vi "Settings Dialog.vi"(8 "error in (no error)":errorcluster, 9 "UI State":T1, 10 "Message Queues":T2, 11 "PRM State Cluster In":T6={"PRM Config"={"GUID"="", "Drop Coords"={"Horizontal"=0, "Vertical"=0}, "Process Name"="", "Settings"={"Cycle Period"=500.0, "PID 2 Parameters"={"Input Device"=enum."Default", "Output Device"=enum."Default", "Setpoint"=0.0, "PID gains"={"proportional gain (Kc)"=1.0, "integral time (Ti, min)"=0.01, "derivative time (Td, min)"=0.0}, "output range"={"output low"=0.0, "output high"=100.0}}, "Manual Entry"=0.0, "Auto?"=TRUE, "4-20mA Input Settings"={"Input Channel "=0}, "4-20mA Out Settings"={"Output DAQ Task"=""}, "Input Channel Tag Name "=""}, "Settings Load Count"=0}, "State"=enum."Idle", "Start Time"=timestamp(0 s since 1904-01-01), "Current Time"=timestamp(0 s since 1904-01-01), "First Iteration"=FALSE, "Data"={"4-20mA Input"=0.0, "PID 2 Process Variable"=0.0, "PID 2 Output"=0.0, "4-20mA Output"=0.0}} {"PRM Config"."Settings"."PID 2 Parameters"."output range"."output low" format="%.2f"; "PRM Config"."Settings"."PID 2 Parameters"."output range"."output high" min=0.0 max=100.0 format="%.2f"; "PRM Config"."Settings"."PID 2 Parameters"."PID gains"."derivative time (Td, min)" format="%.3f"; "PRM Config"."Settings"."PID 2 Parameters"."PID gains"."integral time (Ti, min)" format="%.3f"; "PRM Config"."Settings"."PID 2 Parameters"."PID gains"."proportional gain (Kc)" format="%.3f"}) -> (0 "error out":errorcluster, 1 "Cancelled?":bool=TRUE, 2 "UI Refresh Needed?":bool, 3 "PRM State Cluster Out":T6={"PRM Config"={"GUID"="", "Drop Coords"={"Horizontal"=0, "Vertical"=0}, "Process Name"="", "Settings"={"Cycle Period"=500.0, "PID 2 Parameters"={"Input Device"=enum."Default", "Output Device"=enum."Default", "Setpoint"=0.0, "PID gains"={"proportional gain (Kc)"=1.0, "integral time (Ti, min)"=0.01, "derivative time (Td, min)"=0.0}, "output range"={"output low"=0.0, "output high"=100.0}}, "Manual Entry"=0.0, "Auto?"=TRUE, "4-20mA Input Settings"={"Input Channel "=0}, "4-20mA Out Settings"={"Output DAQ Task"=""}, "Input Channel Tag Name "=""}, "Settings Load Count"=0}, "State"=enum."Idle", "Start Time"=timestamp(0 s since 1904-01-01), "Current Time"=timestamp(0 s since 1904-01-01), "First Iteration"=FALSE, "Data"={"4-20mA Input"=0.0, "PID 2 Process Variable"=0.0, "PID 2 Output"=0.0, "4-20mA Output"=0.0}} {"PRM Config"."Settings"."PID 2 Parameters"."output range"."output low" format="%.2f"; "PRM Config"."Settings"."PID 2 Parameters"."output range"."output high" min=0.0 max=100.0 format="%.2f"; "PRM Config"."Settings"."PID 2 Parameters"."PID gains"."derivative time (Td, min)" format="%.3f"; "PRM Config"."Settings"."PID 2 Parameters"."PID gains"."integral time (Ti, min)" format="%.3f"; "PRM Config"."Settings"."PID 2 Parameters"."PID gains"."proportional gain (Kc)" format="%.3f"})   [LabVIEW 2018, in "4-20mA Module.lvlib"]
uses:
  4-20mA Module.lvlib
  Controls/4-20mA Module State Cluster.ctl
  Controls/4-20mA Module Config Cluster.ctl
  <vilib>/Utility/miscctls.llb/LVPoint32TypeDef.ctl
  Controls/4-20mA Module Settings Cluster.ctl
  Pressure Transmitter/Pressure Transmitter Device Settings.ctl
  Pressure Reg Module/Pressure Regulator Device Settings.ctl
  Measure Instrument/State Enum.ctl
  Controls/4-20mA Message Queues.ctl
  support/Message Queue/Message Cluster.ctl
  controls/UI State.ctl
  Tag VIs/Tag FGV Operation Enum.ctl
  <vilib>/Utility/miscctls.llb/LVMinMaxIncTypeDef.ctl
  support/Message Queue/Enqueue Message (Single).vi
  Settings/Settings.lvlib
  Pressure Transmitter/Pressure Transmitter Library.lvlib
  Shared Variables/Dynamic Shared Variables.lvlib
  Pressure Reg Module/Pressure Regulator Library.lvlib
  support/Support Library.lvlib
  support/Message Queue/Message Queue.lvlib
  Flow Regulator/Pressure Reg Module/Flow Regulator Library.lvlib
  <vilib>/Utility/xml.llb/Write to XML File(string).vi
  Measure Instrument/Feed Module Engine.lvlib
panel:
  in  "Module Name":string
  in  "Start":bool
  in  "Stop":bool
  in  "Pressure Regulator Configuration":T5={"Cycle Period"=500.0, "PID 2 Parameters"={"Input Device"=enum."Default", "Output Device"=enum."Default", "Setpoint PSIA"=0.0, "PID gains"={"proportional gain (Kc)"=1.0, "integral time (Ti, min)"=0.01, "derivative time (Td, min)"=0.0}, "output range"={"output low"=0.0, "output high"=100.0}}, "Manual PSIA"=0.0, "Auto?"=TRUE, "4-20mA Input Settings"={"Input Channel "=0}, "Out Settings"={"Output DAQ Task"=""}} {"4-20mA Input Settings"."Input Channel" items=["Default", "TT0", "PT0", "PR 1:4-20mA Input", "PR 1:PID2Out", "PR 1:4-20mA Output", "PR 1:Input Device Disconnected", "PR 1:Output Device Disconnected"]; "Manual PSIA" min=0.0 max=50.0; "PID 2 Parameters"."output range"."output low" format="%.2f"; "PID 2 Parameters"."output range"."output high" min=0.0 max=100.0 format="%.2f"; "PID 2 Parameters"."PID gains"."derivative time (Td, min)" format="%.3f"; "PID 2 Parameters"."PID gains"."integral time (Ti, min)" format="%.3f"; "PID 2 Parameters"."PID gains"."proportional gain (Kc)" format="%.3f"}
  in  "Cancel Button":bool
  in  "OK Button":bool
  # "Output Settings"
  # "Input Settings"
  # "Instrument Settings"
  # "Instrument Settings"
  # "Instrument Settings"
  # "Instrument Settings"
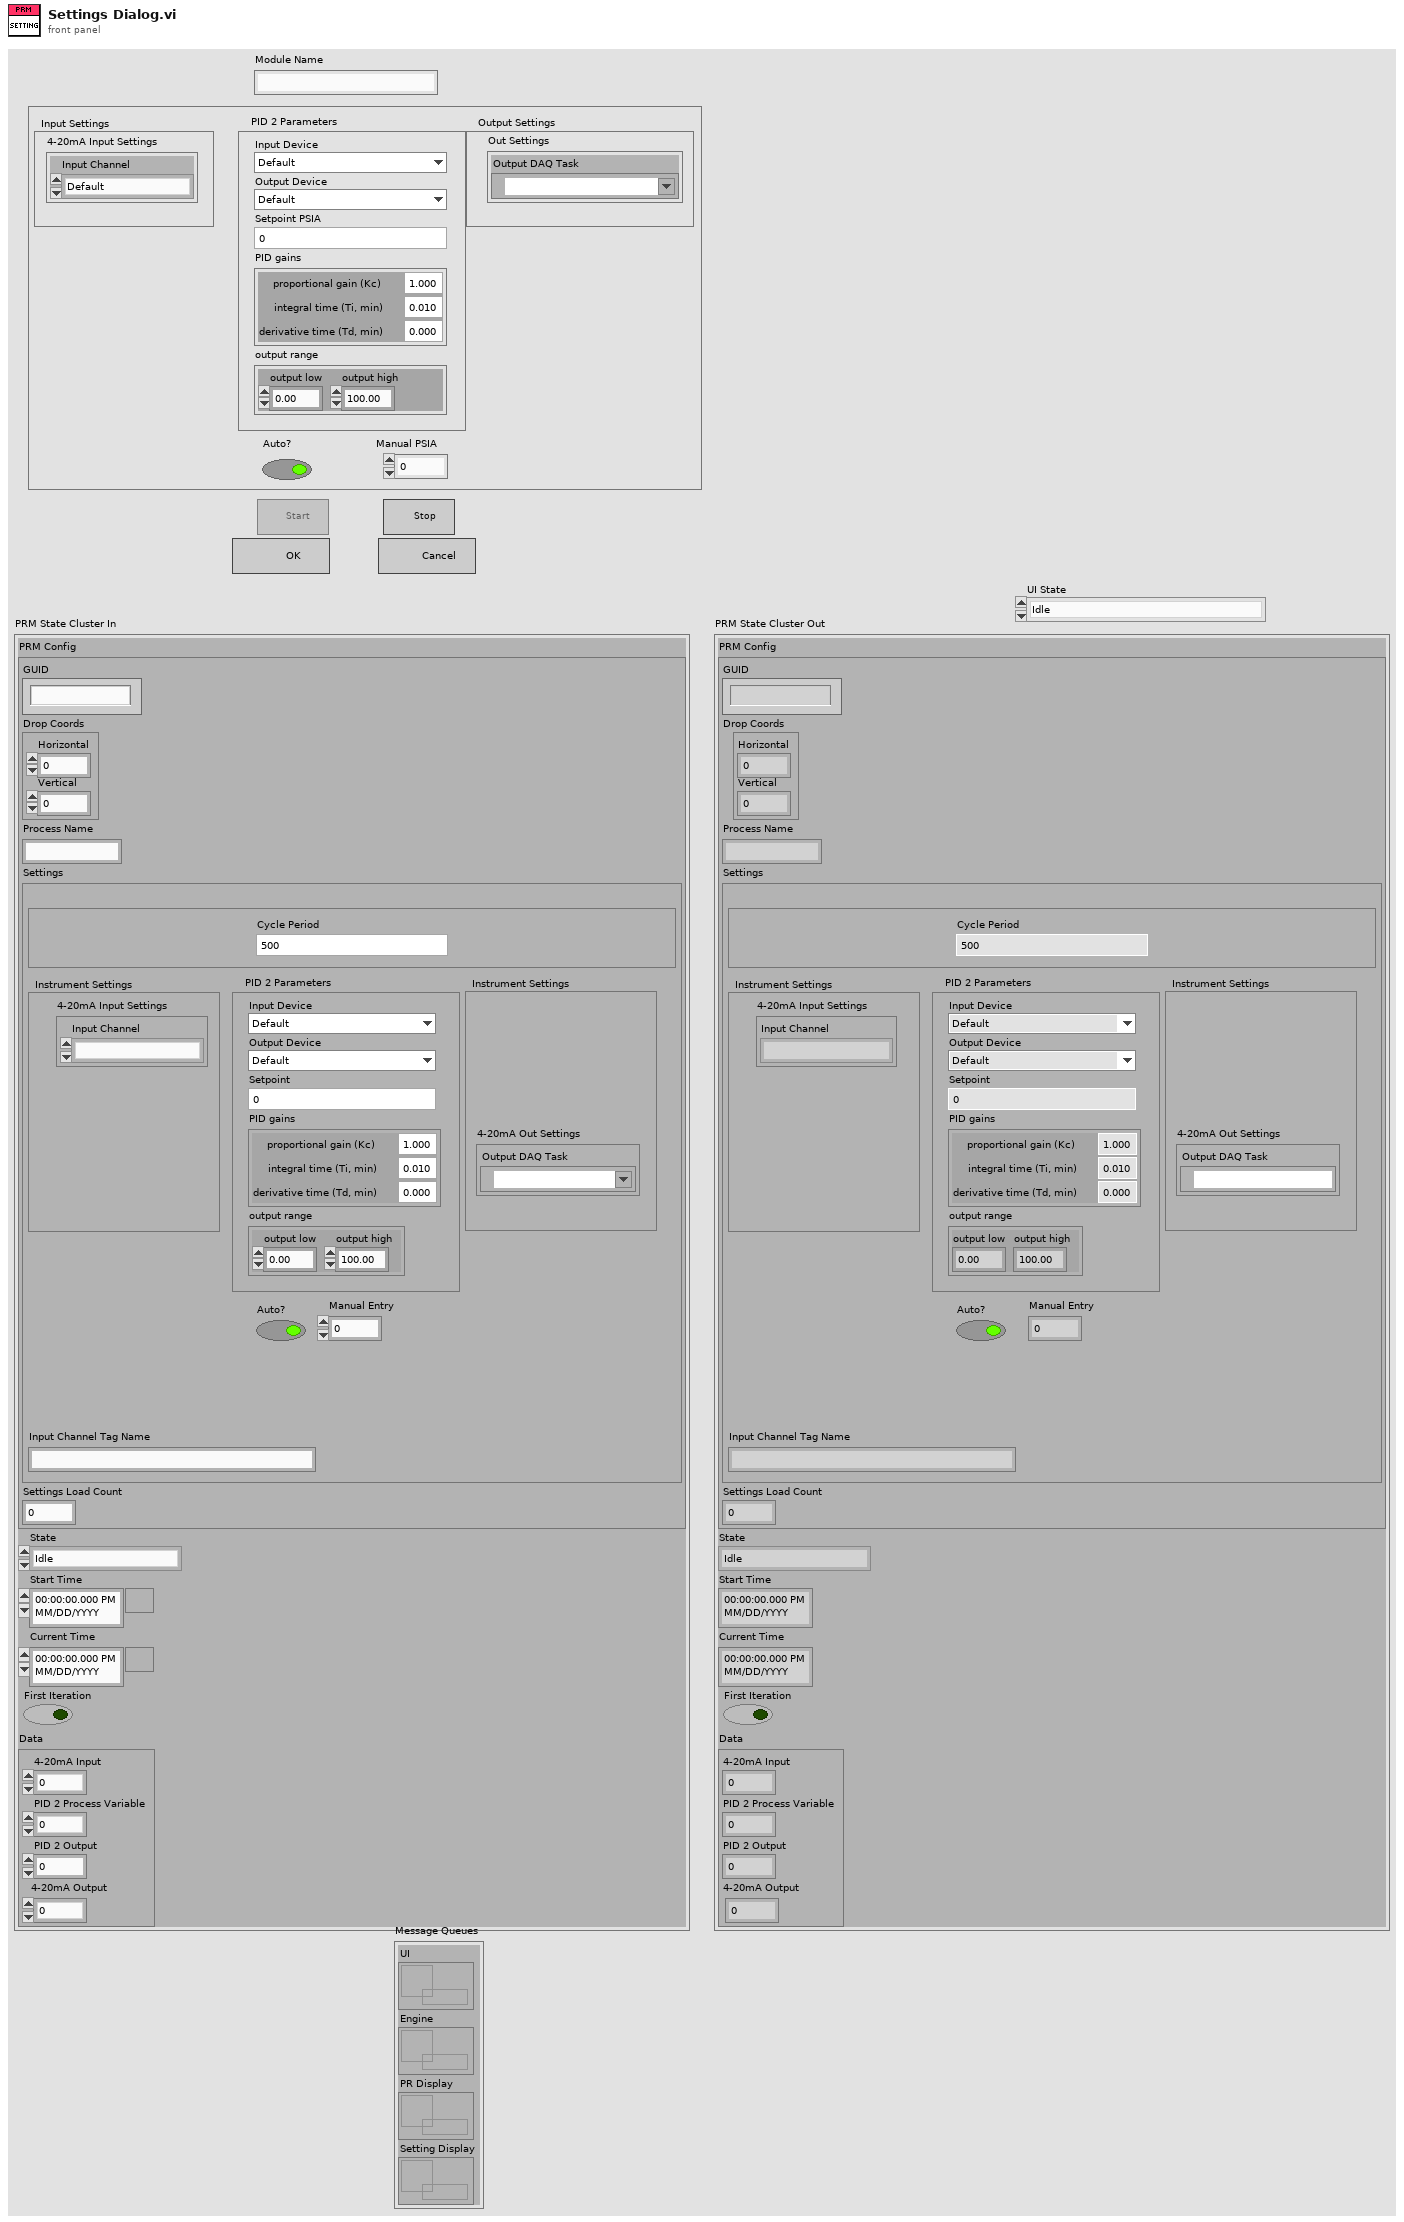
[diagram p1: front panel]
types:
  T1 = typedef "UI State.ctl" = enum16{"Idle", "Acquiring and Logging", "Waiting for Exit", "Waiting for Exit (Acq Stopped)", "Waiting for Exit (Log Stopped)", "Waiting for Stop", "Waiting for Stop (Acq Stopped)", "Waiting for Stop (Log Stopped)"}
  T2 = typedef "4-20mA Module.lvlib/4-20mA Message Queues.ctl" = cluster{"UI":refnum<queue>, "Engine":refnum<queue>, "PR Display":refnum<queue>, "Setting Display":refnum<queue>}
  T3 = typedef "Pressure Transmitter Library.lvlib/Pressure Transmitter Device Settings.ctl" = cluster{"Input Channel ":u16}
  T4 = typedef "Pressure Regulator Library.lvlib/Pressure Regulator Device Settings.ctl" = cluster{"Output DAQ Task":refnum<k21>}
  T5 = cluster{"Cycle Period":dbl, "PID 2 Parameters":cluster{"Input Device":enum16{"Default", "4-20mA"}, "Output Device":enum16{"Default", "Equilibar Pressure Reg", "Flow Regulator"}, "Setpoint PSIA":dbl, "PID gains":cluster{"proportional gain (Kc)":dbl, "integral time (Ti, min)":dbl, "derivative time (Td, min)":dbl}, "output range":cluster{"output low":dbl, "output high":dbl}}, "Manual PSIA":dbl, "Auto?":bool, "4-20mA Input Settings":T3, "Out Settings":T4}
  T6 = typedef "4-20mA Module.lvlib/4-20mA Module State Cluster.ctl" = cluster{"PRM Config":T7, "State":T10, "Start Time":timestamp, "Current Time":timestamp, "First Iteration":bool, "Data":cluster{"4-20mA Input":dbl, "PID 2 Process Variable":dbl, "PID 2 Output":dbl, "4-20mA Output":dbl}}
  T7 = typedef "4-20mA Module.lvlib/4-20mA Module Config Cluster.ctl" = cluster{"GUID":string, "Drop Coords":T8, "Process Name":string, "Settings":T9, "Settings Load Count":i32}
  T8 = typedef "LVPoint32TypeDef.ctl" = cluster{"Horizontal":i32, "Vertical":i32}
  T9 = typedef "4-20mA Module.lvlib/4-20mA Module Settings Cluster.ctl" = cluster{"Cycle Period":dbl, "PID 2 Parameters":cluster{"Input Device":enum16{"Default", "4-20mA"}, "Output Device":enum16{"Default", "Equilibar Pressure Reg", "Flow Regulator"}, "Setpoint":dbl, "PID gains":cluster{"proportional gain (Kc)":dbl, "integral time (Ti, min)":dbl, "derivative time (Td, min)":dbl}, "output range":cluster{"output low":dbl, "output high":dbl}}, "Manual Entry":dbl, "Auto?":bool, "4-20mA Input Settings":T3, "4-20mA Out Settings":T4, "Input Channel Tag Name ":string}
  T10 = typedef "Feed Module.lvlib/Feed Module Engine.lvlib/State Enum.ctl" = enum16{"Measuring", "Idle", "Paused"}
  T11 = typedef "Tag FGV Operation Enum.ctl" = enum16{"Init", "Set Notification Queue", "Create Tag", "Commit", "Write Tag (Numeric)", "Write Tag (Boolean)", "Read All Tags", "Read One Tag", "Delete Tag Category", "Set Alarm Parameters (Numeric)", "Set Alarm Parameters (Boolean)", "Enable All Alarms", "Disable All Alarms", "Delete All Tags", "Read Alarms", "Ack Alarm"}
  T12 = enum8{"Enabled", "Disabled", "Disabled and Grayed Out"}
  T13 = cluster{"Cycle Period":dbl, "PID 2 Parameters":cluster{"Input Device":enum16{"Default", "4-20mA"}, "Output Device":enum16{"Default", "Equilibar Pressure Reg", "Flow Regulator"}, "Setpoint":dbl, "PID gains":cluster{"proportional gain (Kc)":dbl, "integral time (Ti, min)":dbl, "derivative time (Td, min)":dbl}, "output range":cluster{"output low":dbl, "output high":dbl}}, "Manual Entry":dbl, "Auto?":bool, "4-20mA Input Settings":T3, "Out Settings":T4}
  T14 = typedef "LVMinMaxIncTypeDef.ctl" = cluster{"Minimum":dbl, "Maximum":dbl, "Increment":dbl}
  T15 = cluster{"Input Device":enum16{"Default", "4-20mA"}, "Output Device":enum16{"Default", "Equilibar Pressure Reg", "Flow Regulator"}, "Setpoint":dbl, "PID gains":cluster{"proportional gain (Kc)":dbl, "integral time (Ti, min)":dbl, "derivative time (Td, min)":dbl}, "output range":cluster{"output low":dbl, "output high":dbl}}
  T16 = cluster{"Input Device":enum16{"Default", "4-20mA"}, "Output Device":enum16{"Default", "Equilibar Pressure Reg", "Flow Regulator"}, "Setpoint PSIA":dbl, "PID gains":cluster{"proportional gain (Kc)":dbl, "integral time (Ti, min)":dbl, "derivative time (Td, min)":dbl}, "output range":cluster{"output low":dbl, "output high":dbl}}
  T17 = enum16{"Default", "Equilibar Pressure Reg", "Flow Regulator"}
  T18 = cluster{"Numeric Text.Text":dbl, "Numeric Text.Text":dbl, "Numeric Text.Text":dbl}
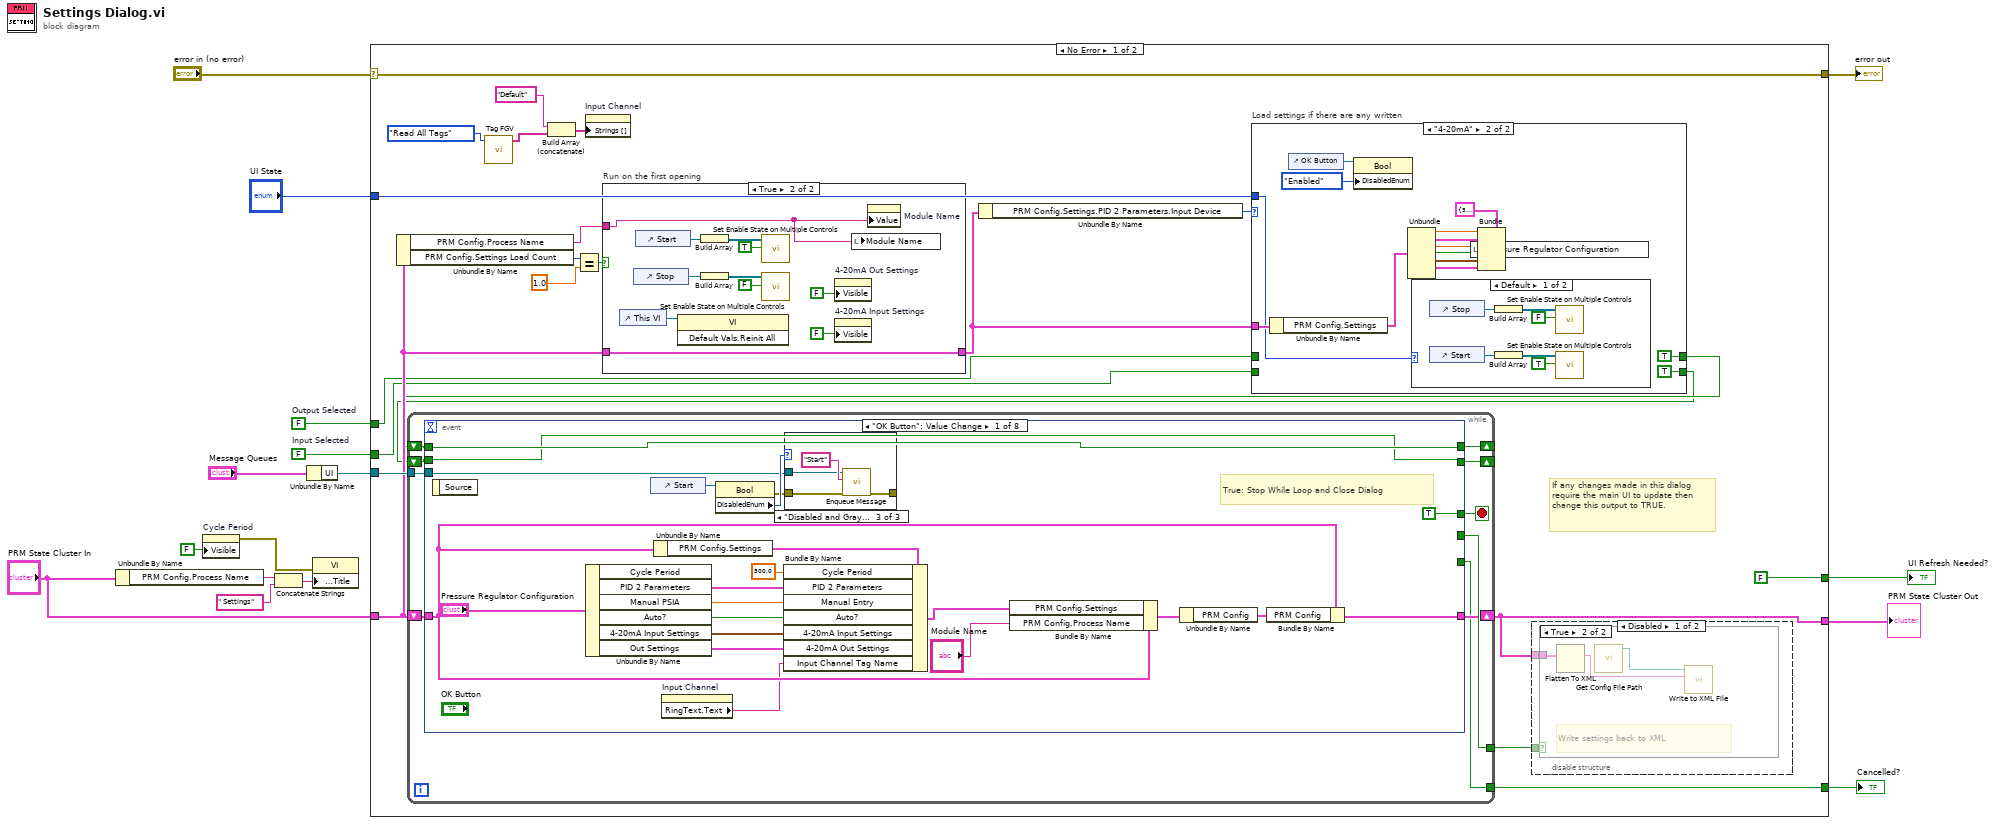
[diagram p0: block diagram]
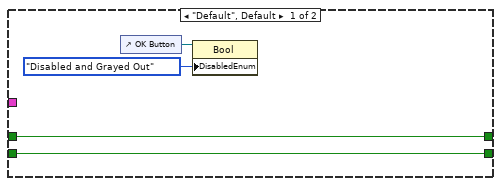
[diagram p4: hidden frame]
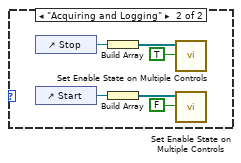
[diagram p5: hidden frame]
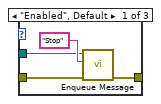
[diagram p7: hidden frame]
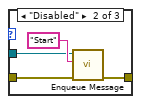
[diagram p8: hidden frame]
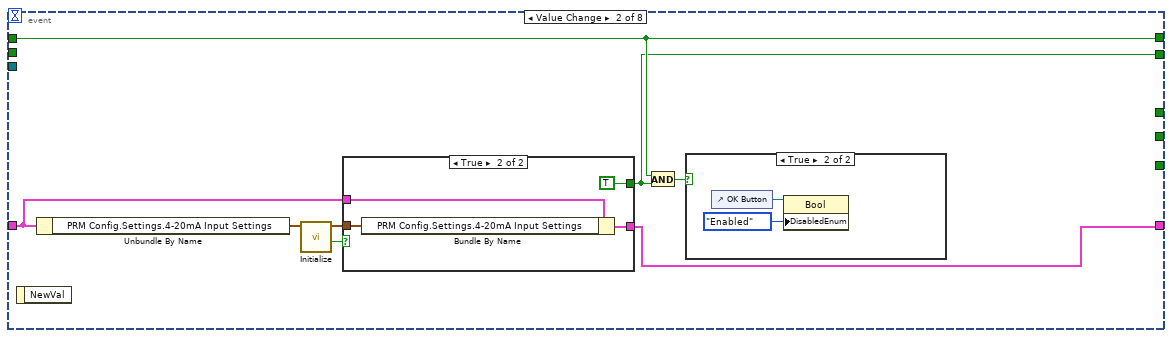
[diagram p9: hidden frame]
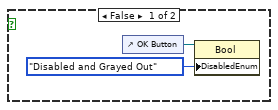
[diagram p10: hidden frame]
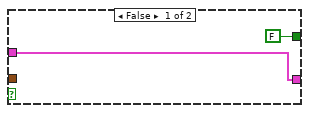
[diagram p11: hidden frame]
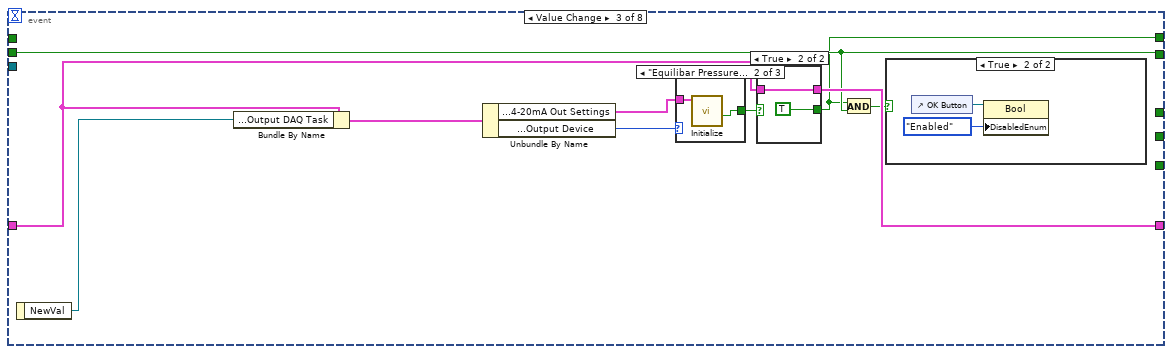
[diagram p12: hidden frame]
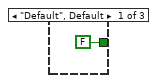
[diagram p13: hidden frame]
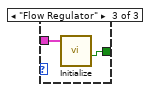
[diagram p14: hidden frame]
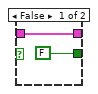
[diagram p15: hidden frame]
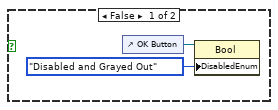
[diagram p16: hidden frame]
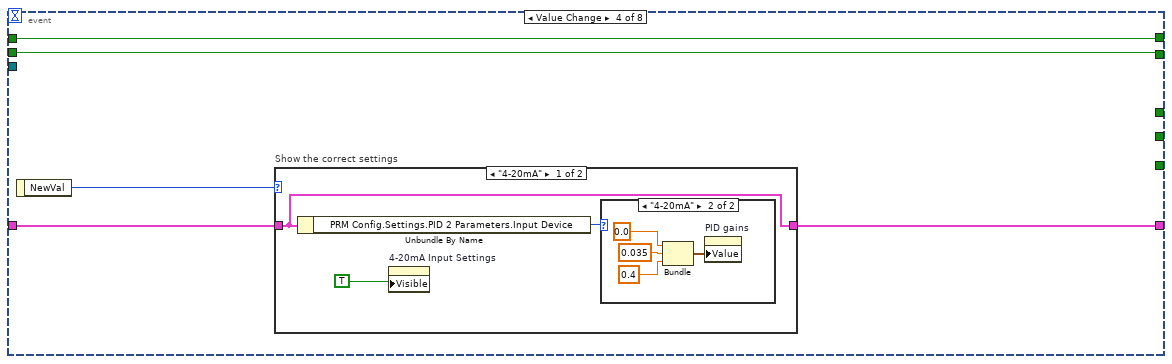
[diagram p17: hidden frame]
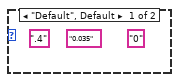
[diagram p18: hidden frame]
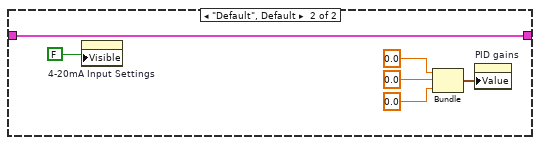
[diagram p19: hidden frame]
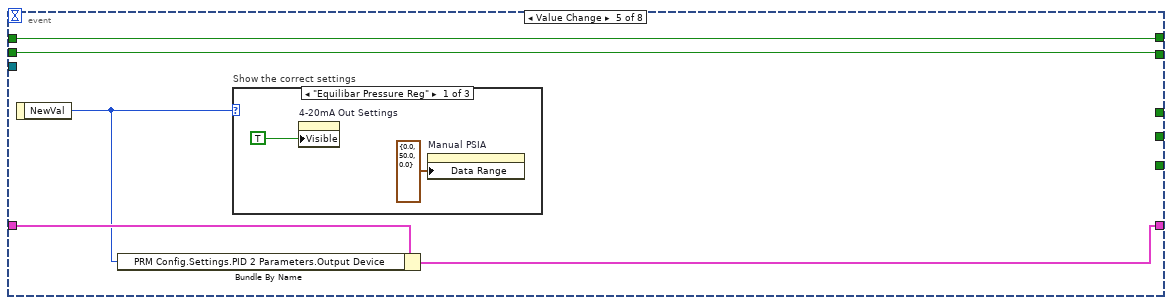
[diagram p20: hidden frame]
diagram:
  w5 = FALSE  # Input Selected
  w6 = FALSE  # Output Selected
  n1 = Unbundle By Name("PRM State Cluster In") -> ("PRM Config.Process Name"=w13:string)
  n2 = property on="Cycle Period" class="DigNum (strict)"("Visible"=FALSE) -> (error out=w1:errorcluster)  [unwired: 2 in, 1 out]
  n3 = Concatenate Strings(w13, " Settings" ("string")) -> (w12:string)
  n4 = Unbundle By Name("Message Queues") -> ("UI"=w7:refnum<queue>)
  n5 = property class="VI"(error in=w1, "Front Panel.Title"=w12) -> ()  [unwired: 1 in, 2 out]
  n6 = case shown="No Error" "error in (no error)" {
    selector: "error in (no error)" -> [w38 w231]
    tunnel: [w38 w231] -> w16
    tunnel: "PRM State Cluster In" -> [w23 w230]
    tunnel: [w36 w230] -> w10
    tunnel: [FALSE ("UI Refresh Needed?") _] -> w15
    tunnel: [w35 TRUE ("UI Refresh Needed?")] -> w14
    tunnel: w7 -> [w24 _]
    tunnel: w6 -> [w22 _]
    tunnel: w5 -> [w21 _]
    tunnel: "UI State" -> [w18 _]
    frame No Error {
      # "If any changes made in this dialog require the main UI to update then change this output to TRUE."
      n7 = Unbundle By Name(w23) -> ("PRM Config.Process Name"=w17:string, "PRM Config.Settings Load Count"=w34:i32)
      n8 = call "Tag FGV.vi"("Operation"=Tag_FGV_Operation_Enum."Read All Tags") -> ("Tag Names"=w26:string[])  [unwired: 5 in, 5 out]
      n9 = Build Array (concatenate)("Default", w26) -> (w25:string[])
      n10 = Equal?(x=w34, y=1.0) -> (x = y?=w31:bool)
      n11 = property on="Input Channel" class="Ring (strict)"("Strings []"=w25) -> ()  [unwired: 2 in, 2 out]
      n12 = case "Run on the first opening" shown="True" w31 {
        tunnel: w23 -> [w75 w85]
        tunnel: [w75 w85] -> w29
        tunnel: w17 -> [_ w76]
        frame False {
        }
        frame True {
          n13 = control-ref of="This VI"() -> (w86:refnum<vi>)
          n14 = control-ref of="Stop"() -> (w81:refnum<vi>)
          n15 = control-ref of="Start"() -> (w82:refnum<vi>)
          n16 = invoke class="VI" method="Default Vals.Reinit All"(reference=w86) -> ()  [unwired: 2 in, 3 out]
          n17 = Build Array(w82) -> (w80:refnum<vi>[])
          n18 = Build Array(w81) -> (w79:refnum<vi>[])
          n19 = call "Set Enable State on Multiple Controls.vi"("Enable?"=TRUE, "Controls"=w80) -> ()  [unwired: 10 in]
          n20 = call "Set Enable State on Multiple Controls.vi"("Enable?"=FALSE, "Controls"=w79) -> ()  [unwired: 10 in]
          n21 = property on="4-20mA Out Settings" class="Clust (strict)"("Visible"=FALSE) -> ()  [unwired: 2 in, 2 out]
          n22 = property on="4-20mA Input Settings" class="Clust (strict)"("Visible"=FALSE) -> ()  [unwired: 2 in, 2 out]
          n23 = local write "Module Name"(w76) -> ()
          n24 = property on="Module Name" class="Str"("Value"=w76) -> ()  [unwired: 2 in, 2 out]
        }
      }
      n25 = Unbundle By Name(w29) -> ("PRM Config.Settings.PID 2 Parameters.Input Device"=w30:enum16{"Default", "4-20mA"})
      n26 = case "Load settings if there are any written" shown="\"4-20mA\"" w30 {
        tunnel: w29 -> [_ w56]
        tunnel: w22 -> [w45 _]
        tunnel: w21 -> [w44 _]
        tunnel: [w45 TRUE] -> w20
        tunnel: [w44 TRUE] -> w19
        tunnel: w18 -> [_ w48]
        frame "Default", Default {
          n27 = control-ref of="OK Button"() -> (w47:refnum<vi>)
          n28 = property on="Property Node" class="Bool"(reference=w47, "DisabledEnum"=T12."Disabled and Grayed Out" ("Disabled")) -> ()  [unwired: 1 in, 2 out]
        }
        frame "4-20mA" {
          n29 = Unbundle By Name(w56) -> ("PRM Config.Settings"=w60:T9)
          n30 = control-ref of="OK Button"() -> (w54:refnum<vi>)
          n31 = property on="Property Node" class="Bool"(reference=w54, "DisabledEnum"=T12."Enabled" ("Disabled")) -> ()  [unwired: 1 in, 2 out]
          n32 = Unbundle(w60) -> ("Cycle Period"=w61:dbl, "PID 2 Parameters"=w62:T15, "Manual Entry"=w57:dbl, "Auto?"=w58:bool, "4-20mA Input Settings"=w59:T3, "4-20mA Out Settings"=w52:T4)  [unwired: 1 out]
          n33 = case shown="Default" w48 {
            frame Default {
              n34 = control-ref of="Stop"() -> (w66:refnum<vi>)
              n35 = control-ref of="Start"() -> (w67:refnum<vi>)
              n36 = Build Array(w66) -> (w65:refnum<vi>[])
              n37 = Build Array(w67) -> (w68:refnum<vi>[])
              n38 = call "Set Enable State on Multiple Controls.vi"("Enable?"=FALSE, "Controls"=w65) -> ()  [unwired: 10 in]
              n39 = call "Set Enable State on Multiple Controls.vi"("Enable?"=TRUE, "Controls"=w68) -> ()  [unwired: 10 in]
            }
            frame "Acquiring and Logging" {
              n40 = control-ref of="Stop"() -> (w72:refnum<vi>)
              n41 = control-ref of="Start"() -> (w73:refnum<vi>)
              n42 = Build Array(w72) -> (w71:refnum<vi>[])
              n43 = Build Array(w73) -> (w74:refnum<vi>[])
              n44 = call "Set Enable State on Multiple Controls.vi"("Enable?"=TRUE, "Controls"=w71) -> ()  [unwired: 10 in]
              n45 = call "Set Enable State on Multiple Controls.vi"("Enable?"=FALSE, "Controls"=w74) -> ()  [unwired: 10 in]
            }
          }
          n46 = Bundle(cluster=T13 {"Cycle Period"=500.0, "PID 2 Parameters"={"Input Device"=enum."Default", "Output Device"=enum."Default", "Setpoint"=0.0, "PID gains"={"proportional gain (Kc)"=1.0, "integral time (Ti, min)"=0.01, "derivative time (Td, min)"=0.0}, "output range"={"output low"=0.0, "output high"=100.0}}, "Manual Entry"=0.0, "Auto?"=TRUE, "4-20mA Input Settings"={"Input Channel "=0}, "Out Settings"={"Output DAQ Task"=""}} ("Configuration"), "Cycle Period"=w61, "PID 2 Parameters"=w62, "Manual Entry"=w57, "Auto?"=w58, "4-20mA Input Settings"=w59, "Out Settings"=w52) -> (w55:T13)
          n47 = local write "Pressure Regulator Configuration"(w55) -> ()
        }
      }
      n48 = while {
        tunnel: [w96] -> w32
        tunnel: [w93] -> w35
        tunnel: w24 -> [w92]
        shift-right: [w88] -> _
        shift-left: w20 -> [w91]
        shift-right: [w89] -> _
        shift-left: w19 -> [w90]
        shift-right: [w95] -> w36
        shift-left: w23 -> [w87]
        stop <- w94 stop-if-true
        n49 = event shown="[0] \"OK Button\": Value Change" {
          selector: _ -> [_ _ _ _ _ _ _ _]
          dyn-events: _ -> [_ _ _ _ _ _ _ _]
          timeout: _ -> [_ _ _ _ _ _ _ _]
          tunnel: [w106 w140 w160 w178 w192 w202 w219 w228] -> w95
          tunnel: w87 -> [w107 w137 w154 w177 w194 w205 w219 w228]
          tunnel: [FALSE ("UI Refresh Needed?") _ _ _ _ FALSE ("UI Refresh Needed?") _ _] -> w96
          tunnel: [TRUE _ _ _ _ TRUE _ _] -> w94
          tunnel: [FALSE ("UI Refresh Needed?") _ _ _ _ TRUE ("UI Refresh Needed?") _ _] -> w93
          tunnel: w92 -> [w102 _ _ _ _ _ _ _]
          tunnel: w91 -> [w100 w134 _ w175 w196 w207 w212 w221]
          tunnel: w90 -> [w99 _ w156 w174 w195 w206 w211 w220]
          tunnel: [w99 w133 w156 w174 w195 w206 w211 w220] -> w89
          tunnel: [w100 w134 w152 w175 w196 w207 w212 w221] -> w88
          event "OK Button": Value Change {
            # "True: Stop While Loop and Close Dialog"
            n50 = event-data() -> ()  [unwired: 1 in, 1 out]
            n51 = Unbundle By Name("Pressure Regulator Configuration") -> ("PID 2 Parameters"=w116:T16, "Manual PSIA"=w115:dbl, "Auto?"=w114:bool, "4-20mA Input Settings"=w112:T3, "Out Settings"=w111:T4)  [unwired: 1 out]
            n52 = control-ref of="Start"() -> (w101:refnum<vi>)
            n53 = Unbundle By Name(w107) -> ("PRM Config.Settings"=w110:T9)
            n54 = property on="Input Channel" class="Ring (strict)"() -> ("RingText.Text"=w105:string)  [unwired: 2 in, 2 out]
            n55 = property class="Bool"(reference=w101) -> (error out=w103:errorcluster, "DisabledEnum"=w104:T12)  [unwired: 1 in, 1 out]
            n56 = Bundle By Name(cluster=w110, "Cycle Period"=500.0, "PID 2 Parameters"=w116, "Manual Entry"=w115, "Auto?"=w114, "4-20mA Input Settings"=w112, "4-20mA Out Settings"=w111, "Input Channel Tag Name"=w105) -> (w113:T9)
            n57 = case shown="\"Disabled and Grayed Out\"" w104 {
              tunnel: w103 -> [w122 w127 w131]
              tunnel: [w124 w126 w130] -> _
              tunnel: w102 -> [w121 w125 w129]
              frame "Enabled", Default {
                n58 = call-poly "Enqueue Message.vi"("error in (no error)"=w122, "Message"="Stop", "Message Queue"=w121) -> ("error out"=w124:errorcluster)  [unwired: 7 in, 1 out]
              }
              frame "Disabled" {
                n59 = call-poly "Enqueue Message.vi"("error in (no error)"=w127, "Message"="Start", "Message Queue"=w125) -> ("error out"=w126:errorcluster)  [unwired: 7 in, 1 out]
              }
              frame "Disabled and Grayed Out" {
                n60 = call-poly "Enqueue Message.vi"("error in (no error)"=w131, "Message"="Start", "Message Queue"=w129) -> ("error out"=w130:errorcluster)  [unwired: 7 in, 1 out]
              }
            }
            n61 = Bundle By Name(cluster=w107, "PRM Config.Settings"=w113, "PRM Config.Process Name"="Module Name") -> (w109:T6)
            n62 = Unbundle By Name(w109) -> ("PRM Config"=w108:T7)
            n63 = Bundle By Name(cluster=w107, "PRM Config"=w108) -> (w106:T6)
          }
          event Value Change {
            n64 = event-data() -> ()  [unwired: 1 in, 1 out]
            n65 = Unbundle By Name(w137) -> ("PRM Config.Settings.4-20mA Input Settings"=w136:T3)
            n66 = call "Initialize.vi"("4-20mA Settings In"=w136) -> ("Initialized"=w139:bool, "4-20mA Settings Out"=w138:T3)  [unwired: 8 in, 1 out]
            n67 = case shown="True" w139 {
              tunnel: w137 -> [w146 w150]
              tunnel: [w146 w148] -> w140
              tunnel: w138 -> [_ w149]
              tunnel: [FALSE TRUE] -> w133
              frame False {
              }
              frame True {
                n68 = Bundle By Name(cluster=w150, "PRM Config.Settings.4-20mA Input Settings"=w149) -> (w148:T6)
              }
            }
            n69 = And(x=w134, y=w133) -> (x .and. y?=w135:bool)
            n70 = case shown="True" w135 {
              frame False {
                n71 = control-ref of="OK Button"() -> (w142:refnum<vi>)
                n72 = property on="Property Node" class="Bool"(reference=w142, "DisabledEnum"=T12."Disabled and Grayed Out" ("Disabled")) -> ()  [unwired: 1 in, 2 out]
              }
              frame True {
                n73 = control-ref of="OK Button"() -> (w144:refnum<vi>)
                n74 = property on="Property Node" class="Bool"(reference=w144, "DisabledEnum"=T12."Enabled" ("Disabled")) -> ()  [unwired: 1 in, 2 out]
              }
            }
          }
          event Value Change {
            n75 = event-data() -> ("NewVal"=w155:refnum<k21>)  [unwired: 1 in]
            n76 = Bundle By Name(cluster=w154, "PRM Config.Settings.4-20mA Out Settings.Output DAQ Task"=w155) -> (w153:T6)
            n77 = Unbundle By Name(w153) -> ("PRM Config.Settings.4-20mA Out Settings"=w159:T4, "PRM Config.Settings.PID 2 Parameters.Output Device"=w151:T17)
            n78 = case shown="\"Equilibar Pressure Reg\"" w151 {
              tunnel: w159 -> [_ w163 w165]
              tunnel: [FALSE ("Initialized") w162 w164] -> w157
              frame "Default", Default {
              }
              frame "Equilibar Pressure Reg" {
                n79 = call "Initialize.vi"("4-20mA Out Settings In"=w163) -> ("Initialized"=w162:bool)  [unwired: 8 in, 2 out]
              }
              frame "Flow Regulator" {
                n80 = call "Initialize.vi"("4-20mA Out Settings In"=w165) -> ("Initialized"=w164:bool)  [unwired: 8 in, 2 out]
              }
            }
            n81 = case shown="True" w157 {
              tunnel: [w167 w168] -> w160
              tunnel: w154 -> [w167 w168]
              tunnel: [FALSE TRUE] -> w152
              frame False {
              }
              frame True {
              }
            }
            n82 = And(x=w152, y=w156) -> (x .and. y?=w158:bool)
            n83 = case shown="True" w158 {
              frame False {
                n84 = control-ref of="OK Button"() -> (w170:refnum<vi>)
                n85 = property on="Property Node" class="Bool"(reference=w170, "DisabledEnum"=T12."Disabled and Grayed Out" ("Disabled")) -> ()  [unwired: 1 in, 2 out]
              }
              frame True {
                n86 = control-ref of="OK Button"() -> (w172:refnum<vi>)
                n87 = property on="Property Node" class="Bool"(reference=w172, "DisabledEnum"=T12."Enabled" ("Disabled")) -> ()  [unwired: 1 in, 2 out]
              }
            }
          }
          event "Pressure Regulator Configuration.PID 2 Parameters.Input Device": Value Change {
            n88 = event-data() -> ("NewVal"=w176:enum16{"Default", "4-20mA"})  [unwired: 1 in]
            n89 = case "Show the correct settings" shown="\"4-20mA\"" w176 {
              tunnel: [w180 w191] -> w178
              tunnel: w177 -> [w180 w191]
              frame "4-20mA" {
                n90 = Unbundle By Name(w180) -> ("PRM Config.Settings.PID 2 Parameters.Input Device"=w181:enum16{"Default", "4-20mA"})
                n91 = property on="4-20mA Input Settings" class="Clust (strict)"("Visible"=TRUE) -> ()  [unwired: 2 in, 2 out]
                n92 = case shown="\"4-20mA\"" w181 {
                  frame "Default", Default {
                    (unwired) "0" ("Numeric Text.Text")
                    (unwired) "0.035" ("Numeric Text.Text")
                    (unwired) ".4" ("Numeric Text.Text")
                  }
                  frame "4-20mA" {
                    n93 = Bundle("Numeric Text.Text"=0.0, "Numeric Text.Text"=0.035, "Numeric Text.Text"=0.4) -> (w182:T18)  [unwired: 1 in]
                    n94 = property on="PID gains" class="Clust (strict)"("Value"=w182) -> ()  [unwired: 2 in, 2 out]
                  }
                }
              }
              frame "Default", Default {
                n95 = property on="4-20mA Input Settings" class="Clust (strict)"("Visible"=FALSE) -> ()  [unwired: 2 in, 2 out]
                n96 = Bundle("Numeric Text.Text"=0.0, "Numeric Text.Text"=0.0, "Numeric Text.Text"=0.0) -> (w189:T18)  [unwired: 1 in]
                n97 = property on="PID gains" class="Clust (strict)"("Value"=w189) -> ()  [unwired: 2 in, 2 out]
              }
            }
          }
          event "Pressure Regulator Configuration.PID 2 Parameters.Output Device": Value Change {
            n98 = event-data() -> ("NewVal"=w193:T17)  [unwired: 1 in]
            n99 = Bundle By Name(cluster=w194, "PRM Config.Settings.PID 2 Parameters.Output Device"=w193) -> (w192:T6)
            n100 = case "Show the correct settings" shown="\"Equilibar Pressure Reg\"" w193 {
              frame "Equilibar Pressure Reg" {
                n101 = property on="4-20mA Out Settings" class="Clust (strict)"("Visible"=TRUE) -> ()  [unwired: 2 in, 2 out]
                n102 = property on="Manual PSIA" class="DigNum (strict)"("Data Range"=T14 {"Minimum"=0.0, "Maximum"=50.0, "Increment"=0.0} ("Data Entry Limits")) -> ()  [unwired: 2 in, 2 out]
              }
              frame "Flow Regulator" {
                n103 = property on="4-20mA Out Settings" class="Clust (strict)"("Visible"=TRUE) -> ()  [unwired: 2 in, 2 out]
                n104 = property on="Manual PSIA" class="DigNum (strict)"("Data Range"=T14 {"Minimum"=0.0, "Maximum"=1000.0, "Increment"=0.0} ("Data Entry Limits")) -> ()  [unwired: 2 in, 2 out]
              }
              frame "Default", Default {
                n105 = property on="4-20mA Out Settings" class="Clust (strict)"("Visible"=FALSE) -> ()  [unwired: 2 in, 2 out]
              }
            }
          }
          event "Cancel Button": Value Change; Panel Close {
            # "True: Stop While Loop and Close Dialog"
            n106 = event-data() -> ()  [unwired: 1 in, 1 out]
            n107 = Unbundle By Name(w205) -> ("PRM Config.Settings Load Count"=w204:i32)
            n108 = Decrement(x=w204) -> (x-1=w203:i32)
            n109 = Bundle By Name(cluster=w205, "PRM Config.Settings Load Count"=w203) -> (w202:T6)
          }
          event "Start": Value Change {
            n110 = event-data() -> ()  [unwired: 1 in, 4 out]
            n111 = control-ref of="Start"() -> (w214:refnum<vi>)
            n112 = control-ref of="Stop"() -> (w213:refnum<vi>)
            n113 = Build Array(w214) -> (w215:refnum<vi>[])
            n114 = Build Array(w213) -> (w218:refnum<vi>[])
            n115 = call "Set Enable State on Multiple Controls.vi"("Enable?"=FALSE, "Controls"=w215) -> ()  [unwired: 10 in]
            n116 = call "Set Enable State on Multiple Controls.vi"("Enable?"=TRUE, "Controls"=w218) -> ()  [unwired: 10 in]
          }
          event "Stop": Value Change {
            n117 = event-data() -> ()  [unwired: 1 in, 4 out]
            n118 = control-ref of="Stop"() -> (w225:refnum<vi>)
            n119 = control-ref of="Start"() -> (w224:refnum<vi>)
            n120 = Build Array(w225) -> (w227:refnum<vi>[])
            n121 = Build Array(w224) -> (w223:refnum<vi>[])
            n122 = call "Set Enable State on Multiple Controls.vi"("Enable?"=FALSE, "Controls"=w227) -> ()  [unwired: 10 in]
            n123 = call "Set Enable State on Multiple Controls.vi"("Enable?"=TRUE, "Controls"=w223) -> ()  [unwired: 10 in]
          }
        }
      }
      n124 = disable-structure shown="Disabled" {
        disable-tunnel: w36 -> [w40 _]
        disable-tunnel: w32 -> [w39 _]
        frame Disabled {
          n125 = case shown="True" w39 {
            tunnel: w40 -> [_ w42]
            frame False {
            }
            frame True {
              # "Write settings back to XML"
              n126 = Flatten To XML(anything=w42) -> (xml string=w41:string)
              n127 = call "Get Config File Path.vi"() -> ("XML File Path"=w43:path)  [unwired: 10 in, 1 out]
              n128 = call-poly <vilib>:"Write to XML File.vi"("XML Input"=w41, "XML File Path"=w43) -> ()  [unwired: 7 in, 3 out]
            }
          }
        }
        frame Enabled {
        }
      }
    }
    frame Error {
    }
  }
  "UI Refresh Needed?" <- w15
  "error out" <- w16
  "Cancelled?" <- w14
  "PRM State Cluster Out" <- w10
